vi "Handle Tree Run Time Menu Item Select.vi"(6 "Coords":T1, 8 "error in (no error)":errorcluster, 9 "ItemPath":string, 10 "ItemTag":string, 11 "Test Executive Explorer in":refnum<class "Test Executive Explorer.lvclass">) -> (0 "error out":errorcluster, 3 "Test Executive Explorer out":refnum<class "Test Executive Explorer.lvclass">)   [LabVIEW 2017, in "Test Executive Explorer.lvclass"]
doc: "<RequiredOverrideReason>The action to take for a given Right-click run time menu selection in the file explorer tree.</RequiredOverrideReason>"
uses:
  Test Executive Explorer.lvclass
  <vilib>/gpm_packages/@cs/file-explorer-extension/Source/File Explorer/File Explorer/File Explorer.lvclass
  Source/Application Dependencies/Create Test Executive.ctl
  Source/Application Dependencies/Create Paramaterized Executive.ctl
  Source/Application Dependencies/Save As Test Executive.ctl
  C:/Users/jonmc/Documents/Git/Test Executive Builder/gpm_packages/@cs/file-explorer-extension/Source/File Explorer/File Explorer/File Explorer.lvclass
  <vilib>/Utility/miscctls.llb/LVPoint32TypeDef.ctl
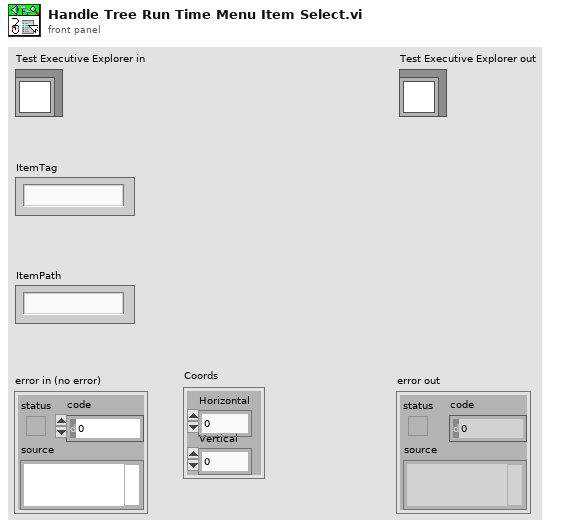
[diagram p1: front panel]
types:
  T1 = typedef "LVPoint32TypeDef.ctl" = cluster{"Horizontal":i32, "Vertical":i32}
  T2 = typedef "Create Test Executive.ctl" = cluster{"Folder Path":path, "File Name with Extension":string}
  T3 = typedef "Create Paramaterized Executive.ctl" = cluster{"Source Folder Path":path, "Source File Name with Extension":string, "Attribute Name Blacklist":string[], "Sink Folder Path":path, "Sink File Name with Extension":string}
  T4 = typedef "Save As Test Executive.ctl" = cluster{"Start Path":path, "Pattern (all files)":string, "Pattern Label":string, "Button Label":string, "Default Name":string, "Prompt":string, "Source File":path, "Delete Source File?":bool}
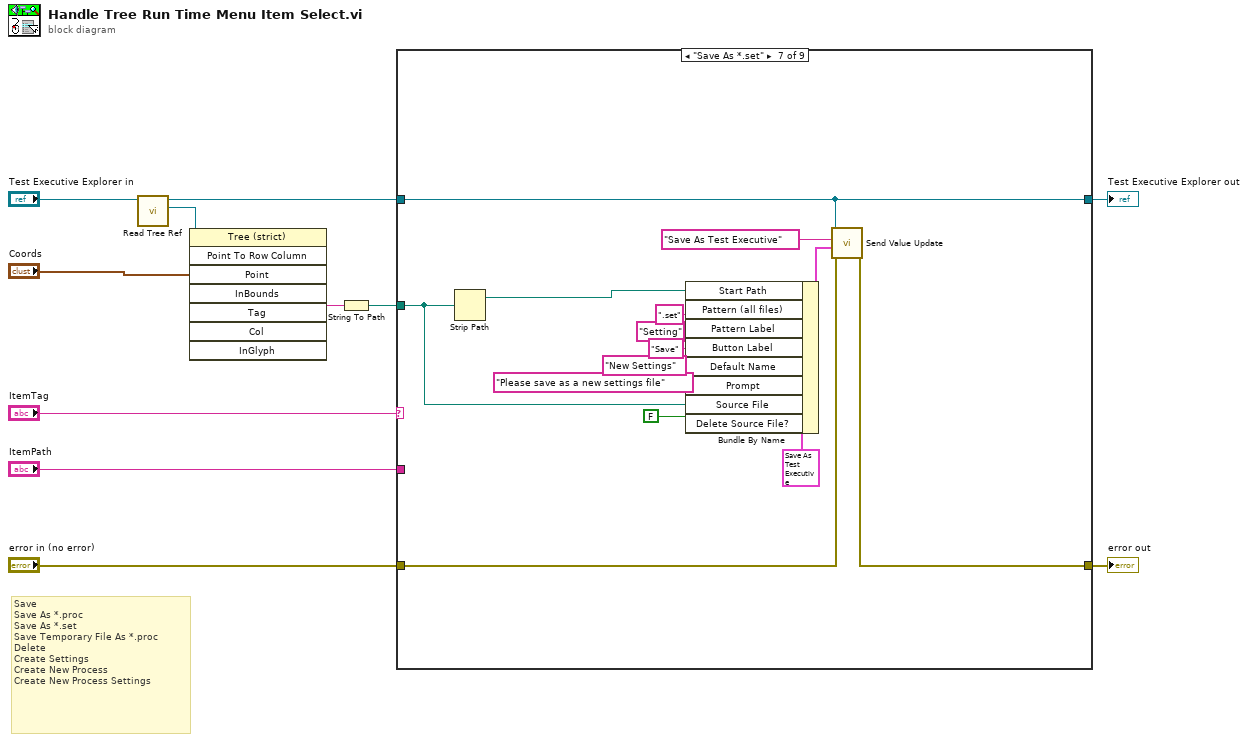
[diagram p0: block diagram]
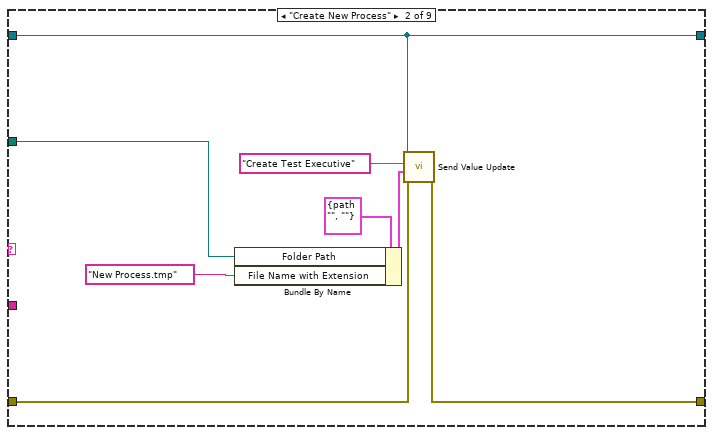
[diagram p3: hidden frame]
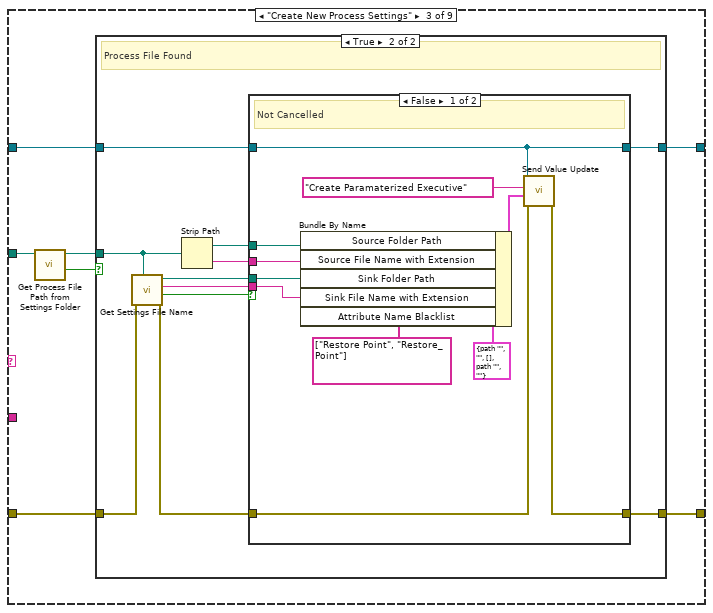
[diagram p4: hidden frame]
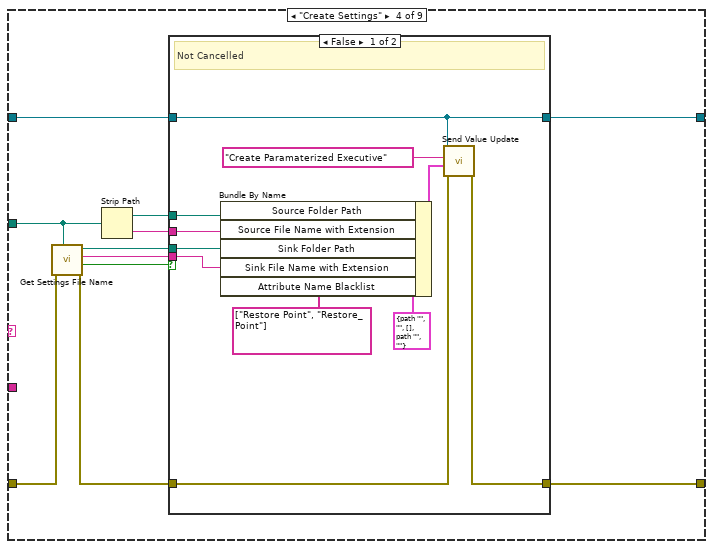
[diagram p7: hidden frame]
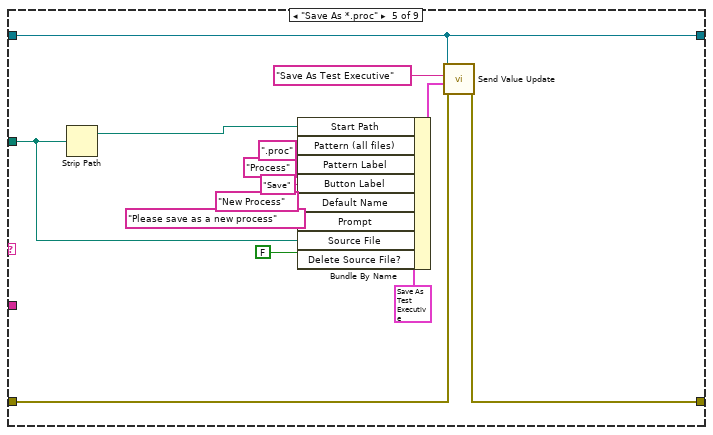
[diagram p9: hidden frame]
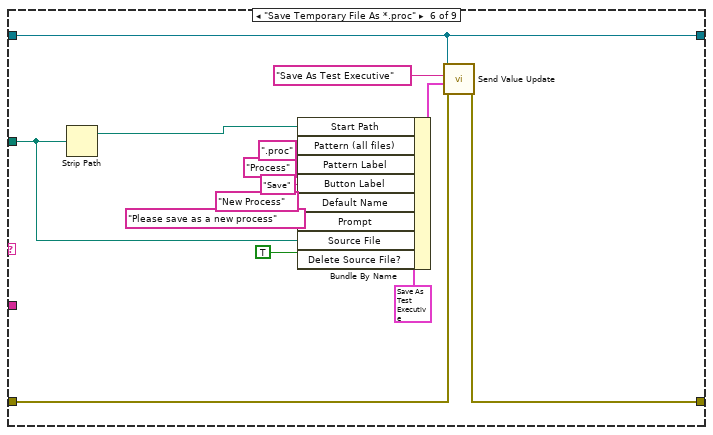
[diagram p10: hidden frame]
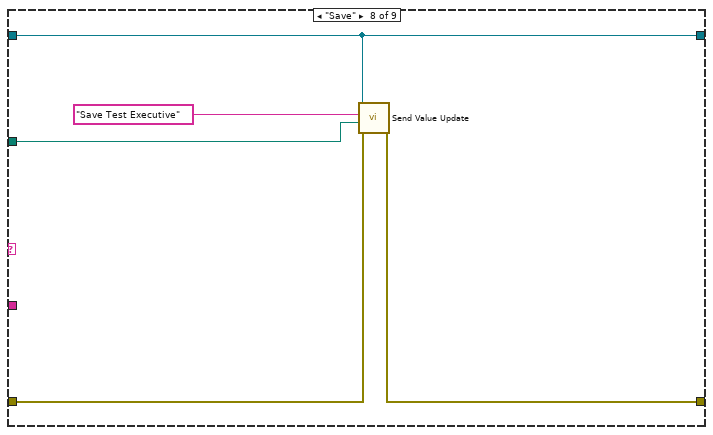
[diagram p11: hidden frame]
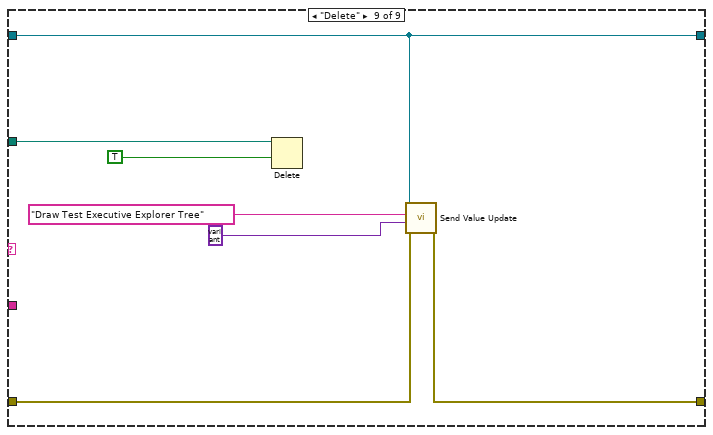
[diagram p12: hidden frame]
diagram:
  # "Save\nSave As *.proc\nSave As *.set\nSave Temporary File As *.proc\nDelete\nCreate Settings\nCreate New Process\nCreate New Process Settings"
  n1 = call <vilib>:"Read Tree Ref.vi"("File Explorer in"="Test Executive Explorer in") -> ("Tree Ref"=w6:refnum<vi>, "File Explorer out"=w4:refnum<class "Test Executive Explorer.lvclass">)  [unwired: 8 in, 1 out]
  n2 = invoke class="Tree (strict)" method="Point To Row Column"(reference=w6, "Point"="Coords") -> ("Tag"=w2:string)  [unwired: 6 in, 7 out]
  n3 = String To Path(string=w2) -> (path=w1:path)
  n4 = case shown="\"Save As *.set\"" "ItemTag" {
    tunnel: "ItemPath" -> [_ _ _ _ _ _ _ _ _]
    tunnel: [w13 w21 w25 w60 w91 w105 w119 w125 w130] -> w9
    tunnel: w4 -> [w13 w21 w28 w65 w91 w105 w119 w125 w130]
    tunnel: [w12 w18 w27 w64 w92 w106 w120 w122 w126] -> w8
    tunnel: "error in (no error)" -> [w12 w19 w26 w63 w90 w104 w118 w123 w127]
    tunnel: w1 -> [_ w15 w24 w61 w85 w99 w113 w121 w132]
    frame Default {
    }
    frame "Create New Process" {
      n5 = Bundle By Name(cluster=T2 {"Folder Path"=path "", "File Name with Extension"=""} ("Create Test Executive"), "Folder Path"=w15, "File Name with Extension"="New Process.tmp") -> (w16:T2)
      n6 = call-dynamic "Send Value Update.vi"("error in (no error)"=w19, "Value"=w16, "Datum Name"="Create Test Executive", "IViewable in"=w21) -> ("error out"=w18:errorcluster)  [unwired: 7 in]
    }
    frame "Create New Process Settings" {
      n7 = call "Get Process File Path from Settings Folder.vi"("Settings Folder"=w24) -> ("Found?"=w22:bool, "Process File Path"=w23:path)  [unwired: 9 in]
      n8 = case shown="True" w22 {
        tunnel: w28 -> [w30 w41]
        tunnel: [w29 w40] -> w27
        tunnel: w26 -> [w29 w39]
        tunnel: w23 -> [_ w37]
        tunnel: [w30 w36] -> w25
        frame False {
          # "Process File Not Found"
        }
        frame True {
          # "Process File Found"
          n9 = call "Get Settings File Name.vi"("Source Path"=w37, "error in (no error)"=w39) -> ("error out"=w38:errorcluster, "Cancelled"=w35:bool, "Sink File"=w32:string, "Sink Folder"=w31:path)  [unwired: 6 in]
          n10 = Strip Path(path=w37) -> (stripped path=w33:path, name=w34:string)
          n11 = case shown="False" w35 {
            tunnel: w41 -> [w47 w54]
            tunnel: [w51 w53] -> w40
            tunnel: w38 -> [w49 w53]
            tunnel: [w47 w54] -> w36
            tunnel: w34 -> [w45 _]
            tunnel: w33 -> [w46 _]
            tunnel: w32 -> [w43 _]
            tunnel: w31 -> [w44 _]
            frame False {
              # "Not Cancelled"
              n12 = Bundle By Name(cluster=T3 {"Source Folder Path"=path "", "Source File Name with Extension"="", "Attribute Name Blacklist"=[], "Sink Folder Path"=path "", "Sink File Name with Extension"=""} ("Create Paramaterized Executive"), "Source Folder Path"=w46, "Source File Name with Extension"=w45, "Sink Folder Path"=w44, "Sink File Name with Extension"=w43, "Attribute Name Blacklist"=string[] ["Restore Point", "Restore_Point"]) -> (w50:T3)
              n13 = call-dynamic "Send Value Update.vi"("error in (no error)"=w49, "Value"=w50, "Datum Name"="Create Paramaterized Executive", "IViewable in"=w47) -> ("error out"=w51:errorcluster)  [unwired: 7 in]
            }
            frame True {
              # "Cancelled"
            }
          }
        }
      }
    }
    frame "Create Settings" {
      n14 = call "Get Settings File Name.vi"("Source Path"=w61, "error in (no error)"=w63) -> ("error out"=w62:errorcluster, "Cancelled"=w59:bool, "Sink File"=w56:string, "Sink Folder"=w55:path)  [unwired: 6 in]
      n15 = Strip Path(path=w61) -> (stripped path=w57:path, name=w58:string)
      n16 = case shown="False" w59 {
        tunnel: w65 -> [w71 w78]
        tunnel: [w75 w77] -> w64
        tunnel: w62 -> [w73 w77]
        tunnel: [w71 w78] -> w60
        tunnel: w58 -> [w69 _]
        tunnel: w57 -> [w70 _]
        tunnel: w56 -> [w67 _]
        tunnel: w55 -> [w68 _]
        frame False {
          # "Not Cancelled"
          n17 = Bundle By Name(cluster=T3 {"Source Folder Path"=path "", "Source File Name with Extension"="", "Attribute Name Blacklist"=[], "Sink Folder Path"=path "", "Sink File Name with Extension"=""} ("Create Paramaterized Executive"), "Source Folder Path"=w70, "Source File Name with Extension"=w69, "Sink Folder Path"=w68, "Sink File Name with Extension"=w67, "Attribute Name Blacklist"=string[] ["Restore Point", "Restore_Point"]) -> (w74:T3)
          n18 = call-dynamic "Send Value Update.vi"("error in (no error)"=w73, "Value"=w74, "Datum Name"="Create Paramaterized Executive", "IViewable in"=w71) -> ("error out"=w75:errorcluster)  [unwired: 7 in]
        }
        frame True {
          # "Cancelled"
        }
      }
    }
    frame "Save As *.proc" {
      n19 = Strip Path(path=w85) -> (stripped path=w86:path)  [unwired: 1 out]
      n20 = Bundle By Name(cluster=T4 {"Start Path"=path "", "Pattern (all files)"="", "Pattern Label"="", "Button Label"="", "Default Name"="", "Prompt"="", "Source File"=path "", "Delete Source File?"=FALSE} ("Save As Test Executive"), "Start Path"=w86, "Pattern (all files)"=".proc", "Pattern Label"="Process", "Button Label"="Save", "Default Name"="New Process", "Prompt"="Please save as a new process", "Source File"=w85, "Delete Source File?"=FALSE) -> (w87:T4)
      n21 = call-dynamic "Send Value Update.vi"("error in (no error)"=w90, "Value"=w87, "Datum Name"="Save As Test Executive", "IViewable in"=w91) -> ("error out"=w92:errorcluster)  [unwired: 7 in]
    }
    frame "Save Temporary File As *.proc" {
      n22 = Strip Path(path=w99) -> (stripped path=w100:path)  [unwired: 1 out]
      n23 = Bundle By Name(cluster=T4 {"Start Path"=path "", "Pattern (all files)"="", "Pattern Label"="", "Button Label"="", "Default Name"="", "Prompt"="", "Source File"=path "", "Delete Source File?"=FALSE} ("Save As Test Executive"), "Start Path"=w100, "Pattern (all files)"=".proc", "Pattern Label"="Process", "Button Label"="Save", "Default Name"="New Process", "Prompt"="Please save as a new process", "Source File"=w99, "Delete Source File?"=TRUE) -> (w101:T4)
      n24 = call-dynamic "Send Value Update.vi"("error in (no error)"=w104, "Value"=w101, "Datum Name"="Save As Test Executive", "IViewable in"=w105) -> ("error out"=w106:errorcluster)  [unwired: 7 in]
    }
    frame "Save As *.set" {
      n25 = Strip Path(path=w113) -> (stripped path=w114:path)  [unwired: 1 out]
      n26 = Bundle By Name(cluster=T4 {"Start Path"=path "", "Pattern (all files)"="", "Pattern Label"="", "Button Label"="", "Default Name"="", "Prompt"="", "Source File"=path "", "Delete Source File?"=FALSE} ("Save As Test Executive"), "Start Path"=w114, "Pattern (all files)"=".set", "Pattern Label"="Setting", "Button Label"="Save", "Default Name"="New Settings", "Prompt"="Please save as a new settings file", "Source File"=w113, "Delete Source File?"=FALSE) -> (w115:T4)
      n27 = call-dynamic "Send Value Update.vi"("error in (no error)"=w118, "Value"=w115, "Datum Name"="Save As Test Executive", "IViewable in"=w119) -> ("error out"=w120:errorcluster)  [unwired: 7 in]
    }
    frame "Save" {
      n28 = call-dynamic "Send Value Update.vi"("error in (no error)"=w123, "Value"=w121, "Datum Name"="Save Test Executive", "IViewable in"=w125) -> ("error out"=w122:errorcluster)  [unwired: 7 in]
    }
    frame "Delete" {
      n29 = Delete(path (use dialog)=w132, confirm (F)=TRUE) -> ()  [unwired: 3 in, 3 out]
      n30 = call-dynamic "Send Value Update.vi"("error in (no error)"=w127, "Value"=variant ("Data Type"), "Datum Name"="Draw Test Executive Explorer Tree", "IViewable in"=w130) -> ("error out"=w126:errorcluster)  [unwired: 7 in]
    }
  }
  "error out" <- w8
  "Test Executive Explorer out" <- w9
